vi "send_receive_command.vi"(0 "reference (in)":i32, 5 "command":T1=enum."get acceleration", 7 "params (opt)":string[](array[string]), 9 "command (raw)":string, 11 "error in (no error)":errorcluster, 12 "echo errors? (T)":bool=TRUE) -> (4 "reference (dup)":i32, 6 "read_string":string, 8 "success?":bool, 10 "write_string":string="ID", 15 "error out":errorcluster)   [LabVIEW 2012]
doc: "Takes as input a reference, command and parameters (optional). The reference input (and passed through as an output) is the reference value for the device that was generated upon initialization. This reference must be included if any device is to be communicated with. Implementss the USB Communication API function \"fnPerformaxComSendRecv\". \n\nThe command is an enumerated constant containing all the commands supported by the LabVIEW USB Communication driver. All commands covered here can be mapped to the commands outlined in the ASCII Language Specification of the USB Communication API documenation.\n\nIf the \"command (raw)\" field is not empty, this VI assumes the user has chosen to send a raw command as outlined in the ASCII Language Specification of the USB Communication API documentation. The \"command\" input field will be ignored.\n\nProduced By:\n\nChristopher Lemieux\nKod Integrations, LLC\n4835 Marianne Drive\nMount Airy, MD 21771\nhttp://www.kodintegrations.com\nemail: clemieux@kodintegrations.com\nphone: (240) 687-1288"
uses:
  commands.ctl
  support/controls/str_array_conv_actions.ctl
  support/controls/errors_actions.ctl
  PerformaxCom.dll
panel:
  in  "pre_init_bytearray":u8[](array[numeric])=[0, 0, 0, 0, 0, 0, 0, 0, 0, 0, 0, 0, 0, 0, 0, 0, 0, 0, 0, 0, 0, 0, 0, 0, 0, 0, 0, 0, 0, 0, 0, 0, 0, 0, 0, 0, 0, 0, 0, 0, 0, 0, 0, 0, 0, 0, 0, 0, 0, 0, 0, 0, 0, 0, 0, 0, 0, 0, 0, 0, 0, 0, 0, 0]
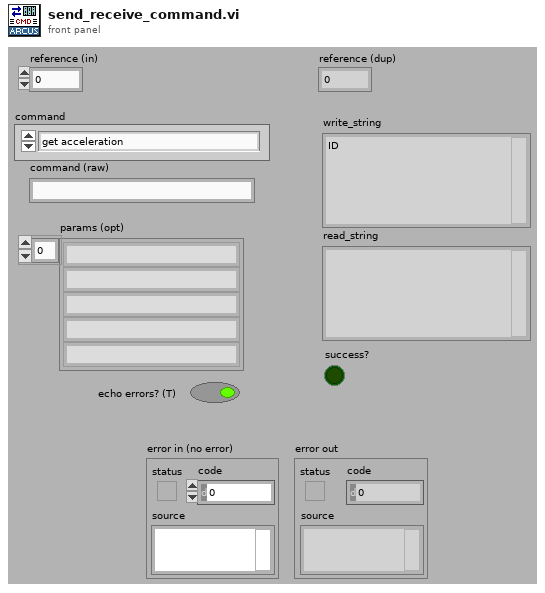
[diagram p1: front panel]
types:
  T1 = typedef "commands.ctl" = enum16{"clear error", "constant jog(-)", "constant jog(+)", "get acceleration", "get actual current", "get device id", "get digital input status", "get digial inputs status", "get dig output status", "get digital outputs status", "get firmware ver", "get high speed", "get idle current", "get low speed", "get micro step", "get motor status", "get move mode", "get polarity", "get position", "get product id", "get power status", "get run current", "get status", "home(-)", "home(+)", "move to position", "power down", "power up", "set acceleration", "set device id", "set digital output", "set digital outputs", "set high speed", "set idle current", "set low speed", "set move mode absolute", "set move mode increment", "set polarity", "set position", "set run current", "stop immediate", "stop slow", "store to memory"}
  T2 = typedef "str_array_conv_actions.ctl" = enum16{"to_bytes", "to_string"}
  T3 = typedef "errors_actions.ctl" = enum16{"clearBuff", "closeRef", "noDeviceInfo", "noDevices", "openRef", "sendReceive", "setTimeouts", "unknown"}
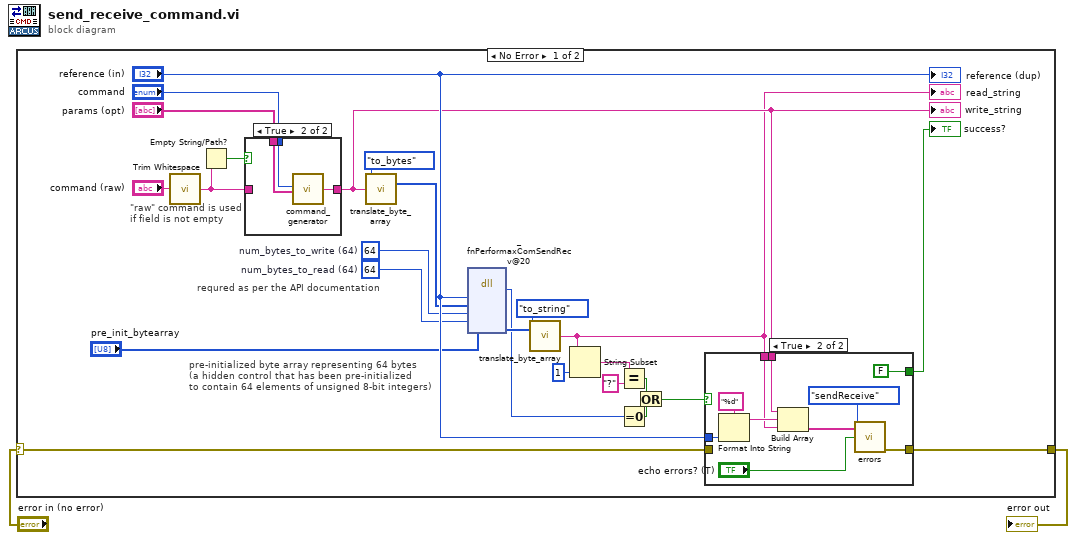
[diagram p0: block diagram]
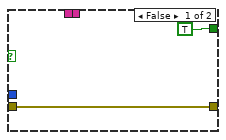
[diagram p3: hidden frame]
diagram:
  n1 = case shown="No Error" "error in (no error)" {
    selector: "error in (no error)" -> [w15 w44]
    tunnel: [w27 w44] -> w1
    frame No Error {
      w20 = 64  # num_bytes_to_write (64)
      w19 = 64  # num_bytes_to_read (64)
      # "\"raw\" command is used\nif field is not empty"
      # "requred as per the API documentation"
      # "pre-initialized byte array representing 64 bytes\n(a hidden control that has been pre-initialized\nto contain 64 elements of unsigned 8-bit integers)"
      n2 = call <vilib>:"Trim Whitespace.vi"("string"="command (raw)") -> ("trimmed string"=w11:string)  [unwired: 1 in]
      n3 = Empty String/Path?(string/path=w11) -> (empty?=w12:bool)
      n4 = case shown="True" w12 {
        tunnel: "command" -> [_ w31]
        tunnel: "params (opt)" -> [_ w30]
        tunnel: [w28 w29] -> w16
        tunnel: w11 -> [w28 _]
        frame False {
        }
        frame True {
          n5 = call "command_generator.vi"("commands"=w31, "args"=w30) -> ("raw_command"=w29:string)  [unwired: 17 in]
        }
      }
      "write_string" <- w16
      n6 = call "translate_byte_array.vi"("actions"=str_array_conv_actions."to_bytes", "string (in)"=w16) -> ("byte_array (out)"=w24:u8[])  [unwired: 12 in, 1 out]
      n7 = dll-call lib="PerformaxCom.dll" fn="_fnPerformaxComSendRecv@20"("reference"="reference (in)", "writeBuffer"=w24, "numBytesToWrite"=w20, "numBytesToRead"=w19, "readBuffer"="pre_init_bytearray") -> (w10:i32, "readBuffer"=w26:u8[])  [unwired: 7 in, 2 out]
      n8 = call "translate_byte_array.vi"("actions"=str_array_conv_actions."to_string", "byte_array (in)"=w26) -> ("string (out)"=w3:string)  [unwired: 12 in, 1 out]
      "read_string" <- w3
      n9 = String Subset(string=w3, length (rest)=1 ("length (rest)")) -> (substring=w4:string)  [unwired: 1 in]
      n10 = Equal?(x=w4, y="?") -> (x = y?=w8:bool)
      n11 = Equal To 0?(x=w10) -> (x = 0?=w7:bool)
      n12 = Or(x=w8, y=w7) -> (x .or. y?=w6:bool)
      n13 = case shown="True" w6 {
        tunnel: [w33 w42] -> w27
        tunnel: w15 -> [w33 _]
        tunnel: "reference (in)" -> [_ w39]
        tunnel: w16 -> [_ w37]
        tunnel: [TRUE FALSE] -> w14
        tunnel: w3 -> [_ w35]
        frame False {
        }
        frame True {
          n14 = Format Into String(format string="%d", w39) -> (resulting string=w38:string)  [unwired: 2 in, 1 out]
          n15 = Build Array(w37, w38, w35) -> (w40:string[])
          n16 = call "errors.vi"("errors"=errors_actions."sendReceive", "dialog? (T)"="echo errors? (T)", "supp_text"=w40) -> ("error out"=w42:errorcluster)  [unwired: 12 in]
        }
      }
      "success?" <- w14
      "reference (dup)" <- "reference (in)"
    }
    frame Error {
    }
  }
  "error out" <- w1
